vi "SFCT heat control tool.vi"() -> ()   [LabVIEW 2020]
uses:
  Desktop/heated tool controller/Status Indicator.ctl
  <vilib>/addons/control/pid/NI_PID_pid.lvlib
panel:
  out "Status":T1
  in  "Tab Control":enum32{"Heat Control", "Motor control"}(tab)
  out "Waveform Chart":cluster{"Numeric":dbl, "Scalar":dbl}(graph)
  in  "Mode":enum16{"Cooling", "Staging", "Compressing"}(ring)
  in  "stop":bool
  out "Loop Speed":u32
  out "Current Temp Tool 1":dbl(slide) scale=0.0..200.0
  in  "Measurement Designations":cluster{"Channel 0":string, "Text Ring":u16}={"Channel 0"="Z1_Tool", "Text Ring"=0} {"Text Ring" items=["cDAQ3Mod1/ai0"]}
  in  "RUN":bool
  out "Profile Preview":cluster{"X":dbl, "Y":dbl}[](graph)
  in  "Timing":enum16{"Hours", "Minutes", "Seconds"}(ring)=enum."Minutes"
  in  "Profile Selection":enum32{"Custom", "Calibration Cycle"}(tab)
  in  "Custom Profile":cluster{"Time (s)":dbl, "Setpoint (C)":dbl}[](array[cluster])=[{"Time (s)"=0.0, "Setpoint (C)"=20.0}, {"Time (s)"=10.0, "Setpoint (C)"=120.0}, {"Time (s)"=25.0, "Setpoint (C)"=120.0}, {"Time (s)"=95.0, "Setpoint (C)"=50.0}, {"Time (s)"=125.0, "Setpoint (C)"=49.0}, {"Time (s)"=168.0, "Setpoint (C)"=180.0}, {"Time (s)"=288.0, "Setpoint (C)"=180.0}]
  out "Custom Profile 2":cluster{"Time (s)":dbl, "Setpoint (C)":dbl}[](array[cluster])
  in  "PID gains z1":T2={"proportional gain (Kc)"=40.0, "integral time (Ti, min)"=0.1, "derivative time (Td, min)"=0.0}
  out "Array":digitalwaveform[](array[waveform])
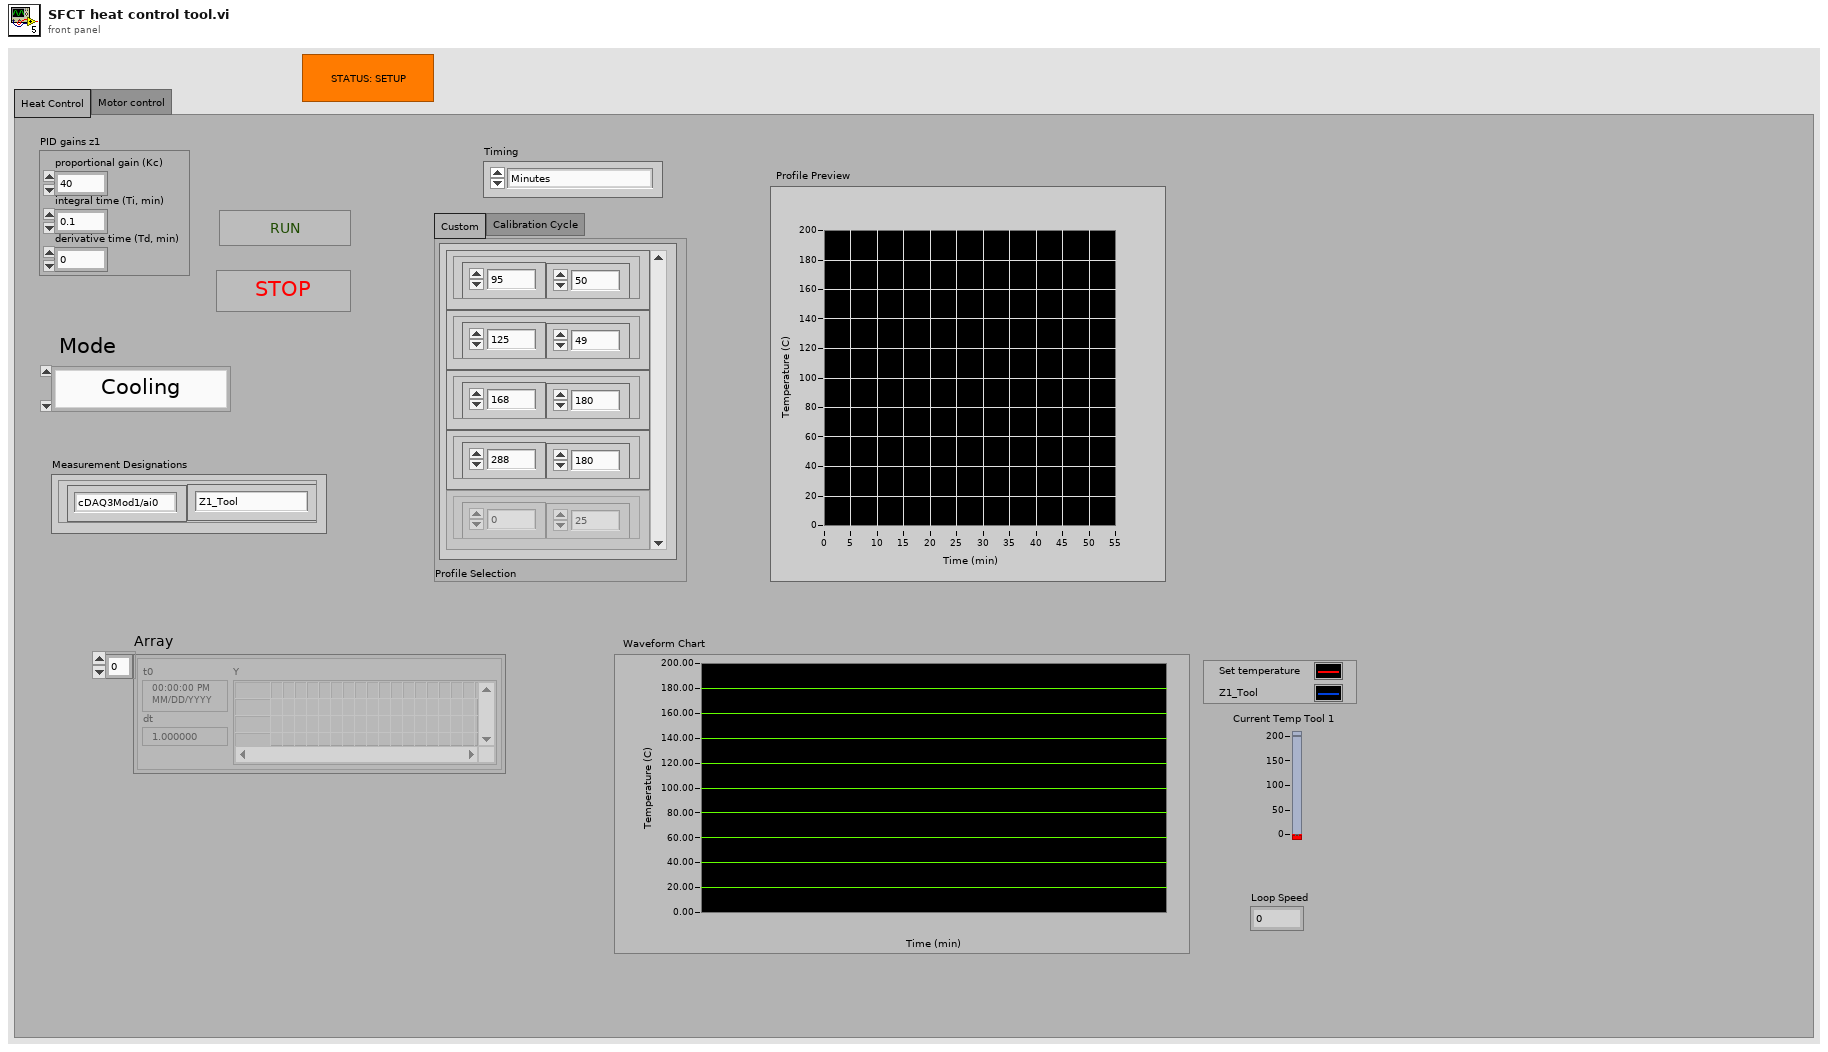
[diagram p1: front panel]
types:
  T1 = typedef "Status Indicator.ctl" = bool
  T2 = cluster{"proportional gain (Kc)":dbl, "integral time (Ti, min)":dbl, "derivative time (Td, min)":dbl}
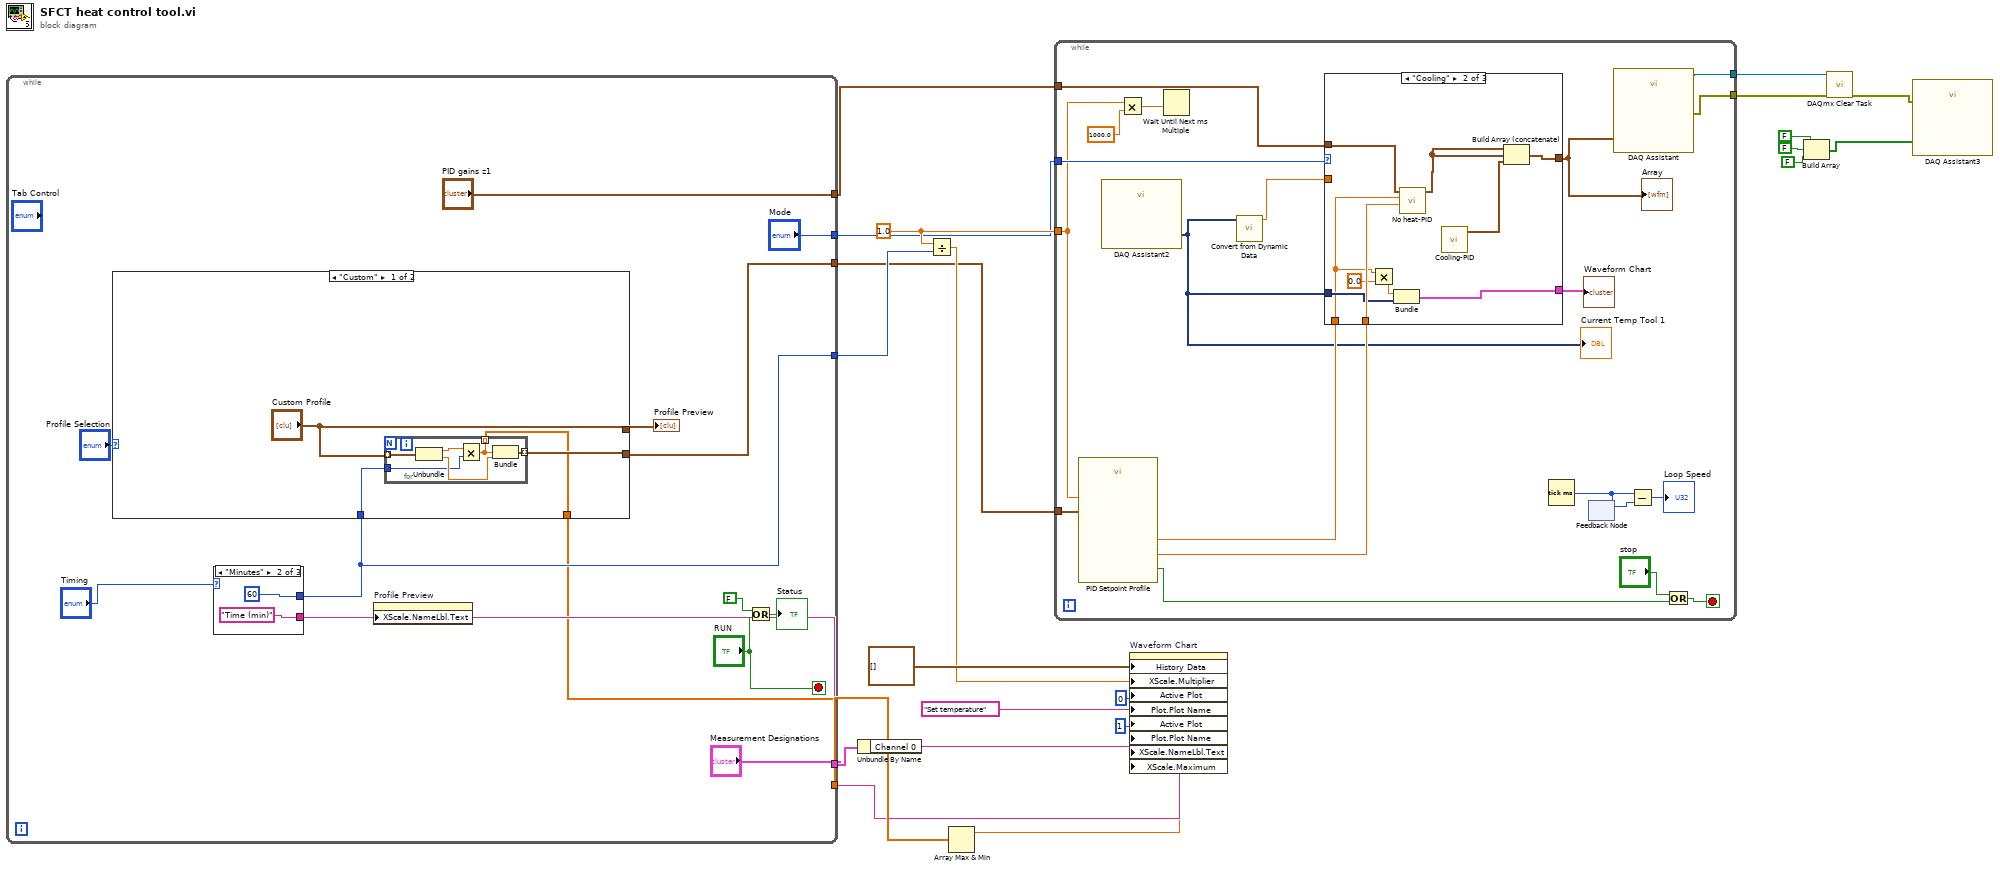
[diagram p0: block diagram]
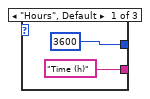
[diagram p2: hidden frame]
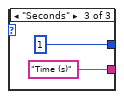
[diagram p3: hidden frame]
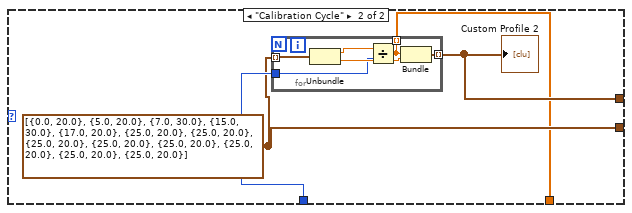
[diagram p4: hidden frame]
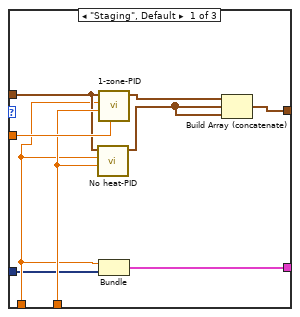
[diagram p5: hidden frame]
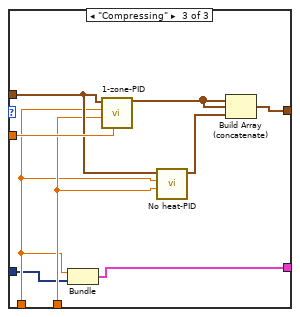
[diagram p6: hidden frame]
diagram:
  w8 = 1.0
  n1 = while {
    tunnel: ["PID gains z1"] -> w6
    tunnel: [w32] -> w7
    tunnel: [w30] -> w19
    tunnel: ["Measurement Designations"] -> w18
    tunnel: [w26] -> w12
    tunnel: [w25] -> w17
    tunnel: ["Mode"] -> w1
    stop <- "RUN" stop-if-true
    n2 = case shown="\"Minutes\"" "Timing" {
      tunnel: [3600 60 1] -> w30
      tunnel: ["Time (h)" "Time (min)" "Time (s)"] -> w26
      frame "Hours", Default {
      }
      frame "Minutes" {
      }
      frame "Seconds" {
      }
    }
    n3 = case shown="\"Custom\"" "Profile Selection" {
      tunnel: [w44 w54] -> w32
      tunnel: w30 -> [w45 w55]
      tunnel: ["Custom Profile" w53] -> w31
      tunnel: [w42 w52] -> w25
      frame "Custom" {
        n4 = for {
          tunnel: "Custom Profile" -> [w51] mode=indexing
          tunnel: [w48] -> w44 mode=indexing
          tunnel: w45 -> [w47]
          tunnel: [w46] -> w42 mode=indexing
          n5 = Unbundle(w51) -> ("Time (s)"=w50:dbl, "Setpoint (C)"=w49:dbl)
          n6 = Multiply(x=w50, y=w47) -> (x*y=w46:dbl)
          n7 = Bundle(w46, "Setpoint (C)"=w49) -> (w48:cluster{dbl, "Setpoint (C)":dbl})  [unwired: 1 in]
        }
      }
      frame "Calibration Cycle" {
        w54 = cluster{"Time (s)":dbl, "Setpoint (C)":dbl}[] [{"Time (s)"=0.0, "Setpoint (C)"=20.0}, {"Time (s)"=5.0, "Setpoint (C)"=20.0}, {"Time (s)"=7.0, "Setpoint (C)"=30.0}, {"Time (s)"=15.0, "Setpoint (C)"=30.0}, {"Time (s)"=17.0, "Setpoint (C)"=20.0}, {"Time (s)"=25.0, "Setpoint (C)"=20.0}, {"Time (s)"=25.0, "Setpoint (C)"=20.0}, {"Time (s)"=25.0, "Setpoint (C)"=20.0}, {"Time (s)"=25.0, "Setpoint (C)"=20.0}, {"Time (s)"=25.0, "Setpoint (C)"=20.0}, {"Time (s)"=25.0, "Setpoint (C)"=20.0}, {"Time (s)"=25.0, "Setpoint (C)"=20.0}, {"Time (s)"=25.0, "Setpoint (C)"=20.0}] ("Custom Profile 2")
        n8 = for {
          tunnel: w54 -> [w61] mode=indexing
          tunnel: [w58] -> w53 mode=indexing
          tunnel: w55 -> [w57]
          tunnel: [w56] -> w52 mode=indexing
          n9 = Unbundle(w61) -> ("Time (s)"=w60:dbl, "Setpoint (C)"=w59:dbl)
          n10 = Divide(x=w60, y=w57) -> (x/y=w56:dbl)
          n11 = Bundle(w56, "Setpoint (C)"=w59) -> (w58:cluster{dbl, "Setpoint (C)":dbl})  [unwired: 1 in]
        }
        "Custom Profile 2" <- w53
      }
    }
    "Profile Preview" <- w31
    n12 = property on="Profile Preview" class="XYGraph (strict)"("XScale.NameLbl.Text"=w26) -> ()  [unwired: 2 in, 2 out]
    n13 = Or(x=FALSE, y="RUN") -> (x .or. y?=→"Status":bool)
  }
  n14 = Unbundle By Name(w18) -> ("Channel 0"=w13:string)
  n15 = Divide(x=w8, y=w19) -> (x/y=w9:dbl)
  n16 = Array Max & Min(array=w17) -> (max value=w11:dbl)  [unwired: 3 out]
  n17 = while {
    tunnel: w1 -> [w81]
    tunnel: [w70] -> w21
    tunnel: [w69] -> w20
    tunnel: w8 -> [w66]
    tunnel: w7 -> [w65]
    tunnel: w6 -> [w64]
    stop <- w76 stop-if-true
    n18 = call <vilib>:"PID Setpoint Profile.vi"("dt (s)"=w66, "setpoint profile"=w65) -> ("dt out (s)"=w79:dbl, "profile complete?"=w77:bool, "setpoint"=w72:dbl)  [unwired: 4 in, 1 out]
    n19 = call "DAQ Assistant2"() -> ("data"=w63:dynamicdata)  [unwired: 17 in, 2 out]
    "Current Temp Tool 1" <- w63
    n20 = Multiply(x=w66, y=1000.0) -> (x*y=w67:dbl)
    n21 = Wait Until Next ms Multiple(millisecond multiple=w67) -> ()  [unwired: 1 out]
    n22 = call "Convert from Dynamic Data"("Dynamic Data Type"=w63) -> ("Scalar"=w71:dbl)  [unwired: 3 in]
    n23 = case shown="\"Cooling\"" w81 {
      tunnel: [w90 w100 w108] -> w80
      tunnel: w79 -> [w88 w97 w104]
      tunnel: w72 -> [w84 w94 w103]
      tunnel: w71 -> [w89 _ w107]
      tunnel: w64 -> [w87 w98 w105]
      tunnel: w63 -> [w83 w95 w102]
      tunnel: [w82 w91 w101] -> w62
      frame "Staging", Default {
        n24 = call "No heat-PID.vi"("dt out (s)"=w88, "setpoint"=w84, "PID gains z1"=w87) -> ("appended array"=w85:digitalwaveform[])  [unwired: 7 in, 1 out]
        n25 = call "1-zone-PID.vi"("Scalar"=w89, "dt out (s)"=w88, "setpoint"=w84, "PID gains z1"=w87) -> ("appended array"=w86:digitalwaveform[])  [unwired: 6 in, 1 out]
        n26 = Bundle("setpoint"=w84, "data"=w83) -> (w82:cluster{"setpoint":dbl, "data":dynamicdata})  [unwired: 1 in]
        n27 = Build Array (concatenate)(w86, w85, w85) -> (w90:digitalwaveform[])
      }
      frame "Cooling" {
        n28 = Multiply(x=w94, y=0.0) -> (x*y=w92:dbl)
        n29 = Bundle(w92, "data"=w95) -> (w91:cluster{dbl, "data":dynamicdata})  [unwired: 1 in]
        n30 = call "No heat-PID.vi"("dt out (s)"=w97, "setpoint"=w94, "PID gains z1"=w98) -> ("appended array"=w99:digitalwaveform[])  [unwired: 7 in, 1 out]
        n31 = call "Cooling-PID.vi"() -> ("appended array"=w96:digitalwaveform[])  [unwired: 11 in]
        n32 = Build Array (concatenate)(w99, w99, w96) -> (w100:digitalwaveform[])
      }
      frame "Compressing" {
        n33 = Bundle("setpoint"=w103, "data"=w102) -> (w101:cluster{"setpoint":dbl, "data":dynamicdata})  [unwired: 1 in]
        n34 = call "1-zone-PID.vi"("Scalar"=w107, "dt out (s)"=w104, "setpoint"=w103, "PID gains z1"=w105) -> ("appended array"=w109:digitalwaveform[])  [unwired: 6 in, 1 out]
        n35 = call "No heat-PID.vi"("dt out (s)"=w104, "setpoint"=w103, "PID gains z1"=w105) -> ("appended array"=w106:digitalwaveform[])  [unwired: 7 in, 1 out]
        n36 = Build Array (concatenate)(w109, w109, w106) -> (w108:digitalwaveform[])
      }
    }
    "Array" <- w80
    "Waveform Chart" <- w62
    n37 = Tick Count (ms)() -> (millisecond timer value=w74:u32)
    n38 = feedback #1() -> (w75:u32)  [unwired: 1 in]
    n39 = feedback-in #1(w74) -> ()
    n40 = call "DAQ Assistant"("data"=w80) -> ("task out"=w70:refnum<k21>, "error out"=w69:errorcluster)  [unwired: 16 in, 1 out]
    n41 = Subtract(x=w74, y=w75) -> (x-y=→"Loop Speed":u32)
    n42 = Or(x="stop", y=w77) -> (x .or. y?=w76:bool)
  }
  n43 = property on="Waveform Chart" class="WFChart (strict)"("History Data"=cluster{"Numeric":dbl, "Scalar":dbl}[] [], "XScale.Multiplier"=w9, "Active Plot"=0, "Plot.Plot Name"="Set temperature", "Active Plot"=1, "Plot.Plot Name"=w13, "XScale.NameLbl.Text"=w12, "XScale.Maximum"=w11) -> ()  [unwired: 2 in, 2 out]
  n44 = Build Array(FALSE, FALSE, FALSE) -> (w3:bool[])
  n45 = call <vilib>:"DAQmx Clear Task.vi"("task in"=w21, "error in"=w20) -> ("error out"=w2:errorcluster)  [unwired: 13 in]
  n46 = call "DAQ Assistant3"("data"=w3, "error in"=w2) -> ()  [unwired: 16 in, 2 out]
